vi "SA Math - ReSample Signals.vi"(0 "Time in":waveform(dbl)[](array[waveform]), 5 "error in (no error)":errorcluster, 6 "Nb Signals":i32, 7 "New Fs":dbl, 8 "Anotate Signal Name":bool=TRUE) -> (14 "Time out":waveform(dbl)[](array[waveform]), 19 "error out":errorcluster)   [LabVIEW 2020, in "GSwFormDSP.lvclass"]
uses:
  GSwFormDSP.lvclass
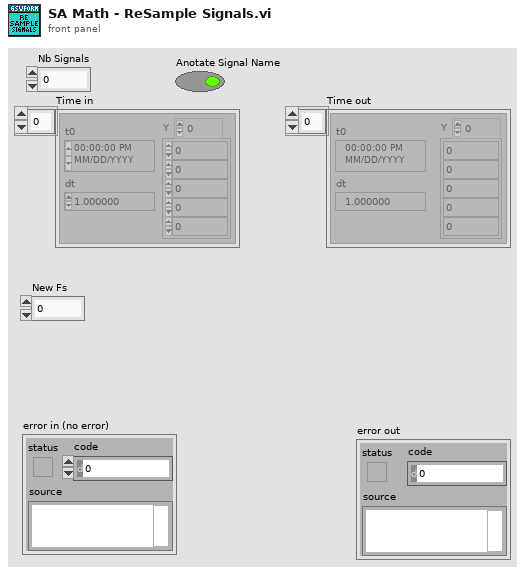
[diagram p1: front panel]
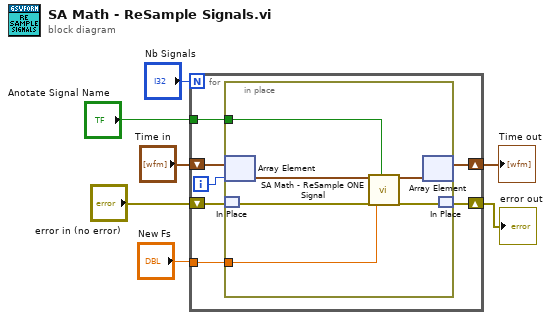
[diagram p0: block diagram]
diagram:
  n1 = for {
    N: "Nb Signals" -> [_]
    shift-right: [w12] -> w5
    shift-left: "Time in" -> [w14]
    shift-right: [w10] -> w6
    shift-left: "error in (no error)" -> [w11]
    tunnel: "New Fs" -> [w9]
    tunnel: "Anotate Signal Name" -> [w8]
    i -> [w13]
    n2 = in-place {
      in-place-border: w9 -> [w17]
      in-place-border: w8 -> [w18]
      n3 = in-place-array #1(w14, w13) -> (w20:waveform(dbl))
      n4 = in-place-match #2(w11) -> (w16:errorcluster)
      n5 = call "SA Math - ReSample ONE Signal.vi"("wForm IN"=w20, "error in (no error)"=w16, "New Fs"=w17, "Anotate Signal Name"=w18) -> ("wForm OUT"=w19:waveform(dbl), "error out"=w15:errorcluster)  [unwired: 13 in, 1 out]
      n6 = in-place-array #1(w19) -> (w12:waveform(dbl)[])  [unwired: 1 out]
      n7 = in-place-match #2(w15) -> (w10:errorcluster)
    }
  }
  "error out" <- w6
  "Time out" <- w5
